vi "Min_Max_and_Average_Value.vi"(0 "SI600.lvclass":refnum<class "SI600.lvclass">, 5 "error in (no error)":errorcluster) -> (10 "RCP Speed Min":dbl, 11 "RCP Speed AVG":dbl, 12 "RCP Speed Max":dbl, 13 "RCP20 Speed":dbl, 14 "SI600.lvclass 2":refnum<class "SI600.lvclass">, 15 "RCP Speed Loop1":dbl, 16 "RCP Speed Loop2":dbl, 17 "RCP Speed Loop3":dbl, 18 "RCP Speed Loop4":dbl, 19 "error IO":errorcluster)   [LabVIEW 2022 SP3, in "SI600.lvclass"]
uses:
  SI600.lvclass
  SI600.lvclass/SI600.ctl
panel:
  in  "Loop40":T1
  in  "Loop30":T2
  in  "Loop20":T3
  in  "Loop10":T4
  # "SI600"
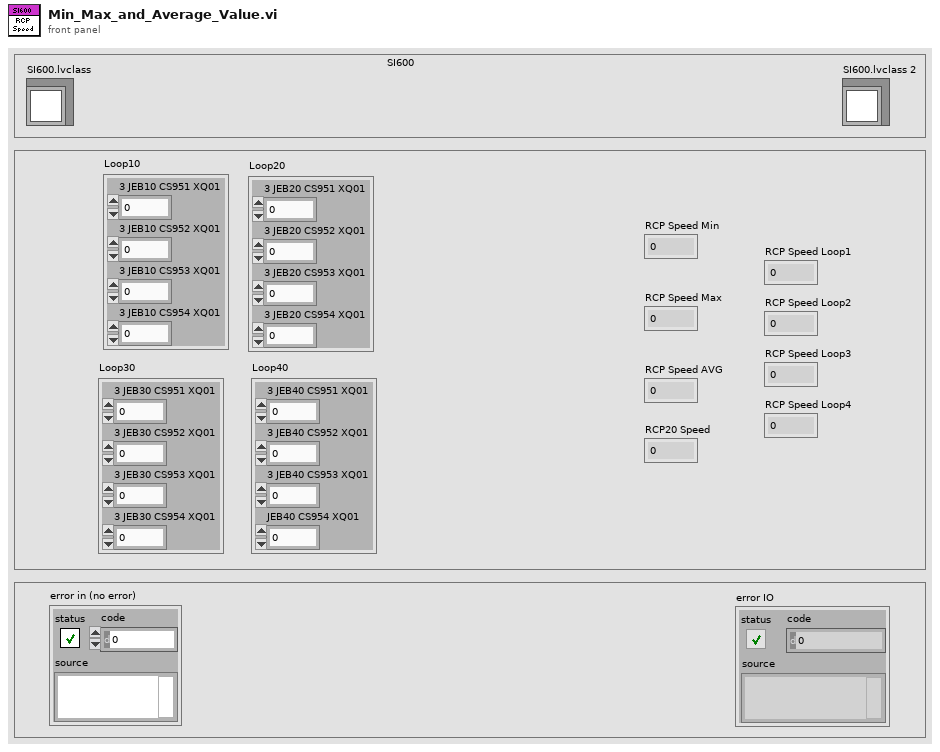
[diagram p1: front panel]
types:
  T1 = cluster{"3 JEB40 CS951 XQ01":dbl, "3 JEB40 CS952 XQ01":dbl, "3 JEB40 CS953 XQ01":dbl, "JEB40 CS954 XQ01":dbl}
  T2 = cluster{"3 JEB30 CS951 XQ01":dbl, "3 JEB30 CS952 XQ01":dbl, "3 JEB30 CS953 XQ01":dbl, "3 JEB30 CS954 XQ01":dbl}
  T3 = cluster{"3 JEB20 CS951 XQ01":dbl, "3 JEB20 CS952 XQ01":dbl, "3 JEB20 CS953 XQ01":dbl, "3 JEB20 CS954 XQ01":dbl}
  T4 = cluster{"3 JEB10 CS951 XQ01":dbl, "3 JEB10 CS952 XQ01":dbl, "3 JEB10 CS953 XQ01":dbl, "3 JEB10 CS954 XQ01":dbl}
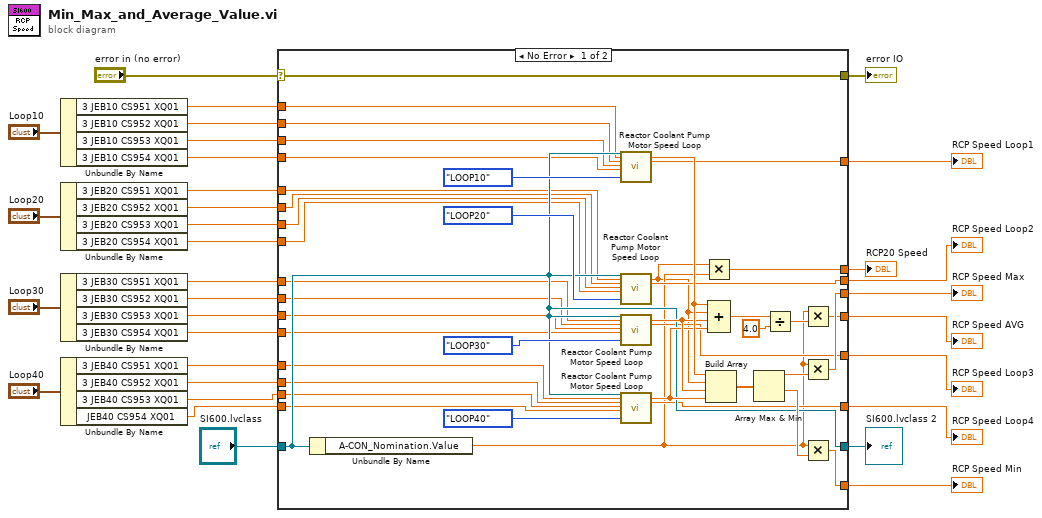
[diagram p0: block diagram]
diagram:
  n1 = Unbundle By Name("Loop10") -> ("3 JEB10 CS951 XQ01"=w18:dbl, "3 JEB10 CS952 XQ01"=w17:dbl, "3 JEB10 CS953 XQ01"=w16:dbl, "3 JEB10 CS954 XQ01"=w15:dbl)
  n2 = Unbundle By Name("Loop20") -> ("3 JEB20 CS951 XQ01"=w14:dbl, "3 JEB20 CS952 XQ01"=w13:dbl, "3 JEB20 CS953 XQ01"=w12:dbl, "3 JEB20 CS954 XQ01"=w11:dbl)
  n3 = Unbundle By Name("Loop30") -> ("3 JEB30 CS951 XQ01"=w9:dbl, "3 JEB30 CS952 XQ01"=w8:dbl, "3 JEB30 CS953 XQ01"=w7:dbl, "3 JEB30 CS954 XQ01"=w6:dbl)
  n4 = Unbundle By Name("Loop40") -> ("3 JEB40 CS951 XQ01"=w4:dbl, "3 JEB40 CS952 XQ01"=w3:dbl, "3 JEB40 CS953 XQ01"=w2:dbl, "JEB40 CS954 XQ01"=w1:dbl)
  n5 = case shown="No Error" "error in (no error)" {
    selector: "error in (no error)" -> [w58 w75]
    tunnel: "SI600.lvclass" -> [w57 w74]
    tunnel: [w61 _] -> w29
    tunnel: [w60 _] -> w30
    tunnel: [w59 _] -> w28
    tunnel: [w58 w75] -> w27
    tunnel: [w57 w74] -> w26
    tunnel: [w56 _] -> w25
    tunnel: [w55 _] -> w24
    tunnel: [w54 _] -> w23
    tunnel: [w53 _] -> w22
    tunnel: [w50 _] -> w21
    tunnel: w18 -> [w49 _]
    tunnel: w17 -> [w48 _]
    tunnel: w16 -> [w47 _]
    tunnel: w15 -> [w46 _]
    tunnel: w14 -> [w45 _]
    tunnel: w13 -> [w44 _]
    tunnel: w12 -> [w43 _]
    tunnel: w11 -> [w42 _]
    tunnel: w9 -> [w41 _]
    tunnel: w8 -> [w40 _]
    tunnel: w7 -> [w39 _]
    tunnel: w6 -> [w38 _]
    tunnel: w4 -> [w36 _]
    tunnel: w3 -> [w35 _]
    tunnel: w2 -> [w34 _]
    tunnel: w1 -> [w33 _]
    frame No Error {
      n6 = Unbundle By Name(w57) -> ("A-CON_Nomination.Value"=w52:dbl)
      n7 = call "Reactor Coolant Pump Motor Speed Loop.vi"("SI600.lvclass in"=w57, "3 JEB CS951 XQ01"=w49, "3 JEB CS952 XQ01"=w48, "3 JEB CS953 XQ01"=w47, "3 JEB CS954 XQ01"=w46, "Loop"=enum16{"LOOP10", "LOOP20", "LOOP30", "LOOP40"}."LOOP10") -> ("RCP speed Loop Output"=w69:dbl, "3 JEB CS951"=w56:dbl)  [unwired: 15 in, 5 out]
      n8 = call "Reactor Coolant Pump Motor Speed Loop.vi"("SI600.lvclass in"=w57, "3 JEB CS951 XQ01"=w45, "3 JEB CS952 XQ01"=w44, "3 JEB CS953 XQ01"=w43, "3 JEB CS954 XQ01"=w42, "Loop"=enum16{"LOOP10", "LOOP20", "LOOP30", "LOOP40"}."LOOP20") -> ("RCP speed Loop Output"=w51:dbl, "3 JEB CS951"=w55:dbl)  [unwired: 15 in, 5 out]
      n9 = call "Reactor Coolant Pump Motor Speed Loop.vi"("SI600.lvclass in"=w57, "3 JEB CS951 XQ01"=w41, "3 JEB CS952 XQ01"=w40, "3 JEB CS953 XQ01"=w39, "3 JEB CS954 XQ01"=w38, "Loop"=enum16{"LOOP10", "LOOP20", "LOOP30", "LOOP40"}."LOOP30") -> ("RCP speed Loop Output"=w68:dbl, "3 JEB CS951"=w54:dbl)  [unwired: 15 in, 5 out]
      n10 = call "Reactor Coolant Pump Motor Speed Loop.vi"("SI600.lvclass in"=w57, "3 JEB CS951 XQ01"=w36, "3 JEB CS952 XQ01"=w35, "3 JEB CS953 XQ01"=w34, "3 JEB CS954 XQ01"=w33, "Loop"=enum16{"LOOP10", "LOOP20", "LOOP30", "LOOP40"}."LOOP40") -> ("RCP speed Loop Output"=w67:dbl, "3 JEB CS951"=w53:dbl)  [unwired: 15 in, 5 out]
      n11 = Multiply(x=w51, y=w52) -> (x*y=w50:dbl)
      n12 = Build Array(w69, w51, w68, w67) -> (w66:dbl[])
      n13 = Compound Arithmetic op=ADD(w69, w51, w68, w67) -> (w70:dbl)
      n14 = Array Max & Min(array=w66) -> (max value=w64:dbl, min value=w63:dbl)  [unwired: 2 out]
      n15 = Divide(x=w70, y=4.0) -> (x/y=w62:dbl)
      n16 = Multiply(x=w52, y=w62) -> (x*y=w59:dbl)
      n17 = Multiply(x=w52, y=w64) -> (x*y=w61:dbl)
      n18 = Multiply(x=w52, y=w63) -> (x*y=w60:dbl)
    }
    frame Error {
    }
  }
  "RCP Speed Min" <- w30
  "RCP Speed Max" <- w29
  "RCP Speed AVG" <- w28
  "error IO" <- w27
  "SI600.lvclass 2" <- w26
  "RCP Speed Loop1" <- w25
  "RCP Speed Loop2" <- w24
  "RCP Speed Loop3" <- w23
  "RCP Speed Loop4" <- w22
  "RCP20 Speed" <- w21
